vi "Serialize - Text.vi"(8 "error in":errorcluster, 11 "Alicat Data in":refnum<class "Alicat Data.lvclass">) -> (0 "error out":errorcluster, 2 "Serialized Text":string, 3 "Alicat Data out":refnum<class "Alicat Data.lvclass">)   [LabVIEW 2015, in "Alicat Lib.lvlib" / "Alicat Data.lvclass"]
uses:
  Alicat Data.lvclass
  Alicat Data.lvclass/Alicat Data.ctl
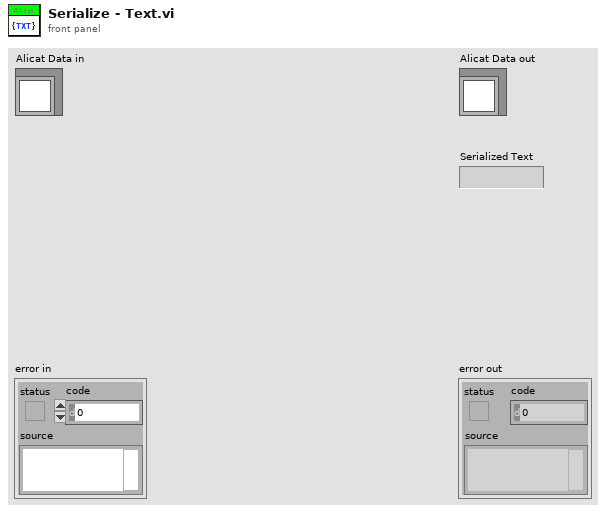
[diagram p1: front panel]
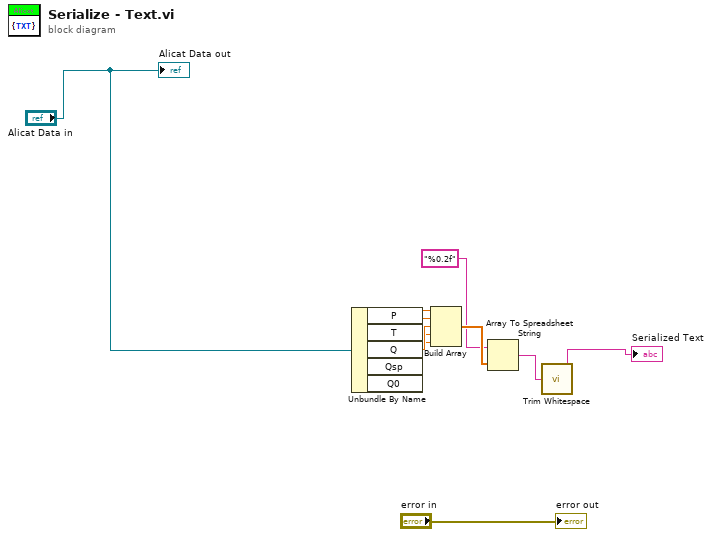
[diagram p0: block diagram]
diagram:
  n1 = Unbundle By Name("Alicat Data in") -> ("P"=w10:sgl, "T"=w9:sgl, "Q"=w8:sgl, "Qsp"=w7:sgl, "Q0"=w6:sgl)
  n2 = Build Array(w10, w9, w8, w7, w6) -> (w5:sgl[])
  n3 = Array To Spreadsheet String(array=w5, 3:"%0.2f" ("format string")) -> (spreadsheet string=w3:string)  [unwired: 1 in]
  n4 = call <vilib>:"Trim Whitespace.vi"("string"=w3) -> ("trimmed string"=→"Serialized Text":string)  [unwired: 1 in]
  "error out" <- "error in"
  "Alicat Data out" <- "Alicat Data in"
